vi "ref_obj_feedback.vi"(1 "input cluster":T1) -> (0 "destination":i16[][](array[numeric]))   [LabVIEW 2010]
uses:
  lib/MWT.dll
panel:
  out "return type 2":i32
  out "return type":i32
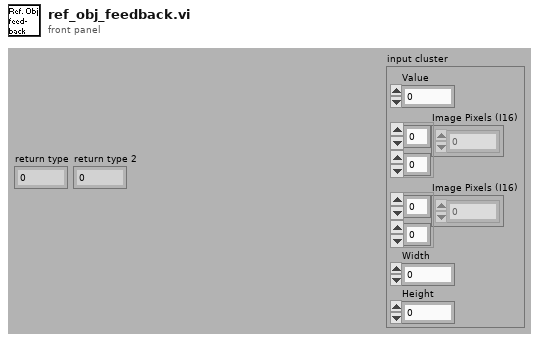
[diagram p1: front panel]
types:
  T1 = cluster{"Value":i32, "Image Pixels (I16)":i16[][], "Image Pixels (I16)":i16[][], "Width":u32, "Height":u32}
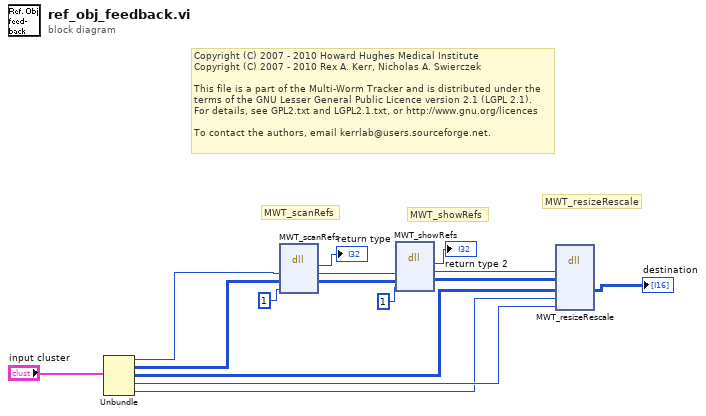
[diagram p0: block diagram]
diagram:
  # "Copyright (C) 2007 - 2010 Howard Hughes Medical Institute\nCopyright (C) 2007 - 2010 Rex A. Kerr, Nicholas A. Swierczek\n \nThis file is a part of the Multi-Worm Tracker and is distributed under the\nterms of the GNU Lesser General Public Licence version 2.1 (LGPL 2.1).\nFor details, see GPL2.txt and LGPL2.1.txt, or http://www.gnu.org/licences\n \nTo contact the authors, email kerrlab@users.sourceforge.net."
  # "MWT_resizeRescale"
  # "MWT_showRefs"
  # "MWT_scanRefs"
  n1 = Unbundle("input cluster") -> ("Value"=w3:i32, "Image Pixels (I16)"=w5:i16[][], "Image Pixels (I16)"=w4:i16[][], "Width"=w2:u32, "Height"=w1:u32)
  n2 = dll-call lib="C:/MWT/lib/MWT.dll" fn="MWT_scanRefs"("handle"=w3, "image"=w5, "bin"=1) -> ("return type"=→"return type":i32, "handle"=w12:i32, "image"=w11:i16[][])  [unwired: 4 in, 2 out]
  n3 = dll-call lib="C:/MWT/lib/MWT.dll" fn="MWT_showRefs"("handle"=w12, "image"=w11, "bin"=1) -> ("return type"=→"return type 2":i32, "handle"=w13:i32, "image"=w14:i16[][])  [unwired: 4 in, 2 out]
  n4 = dll-call lib="C:/MWT/lib/MWT.dll" fn="MWT_resizeRescale"("handle"=w13, "source"=w14, "destination"=w4, "width"=w1, "height"=w2) -> ("destination"=→"destination":i16[][])  [unwired: 8 in, 2 out]
